vi "Aircraft opCRD Server 0.vi"() -> ()   [LabVIEW 2015]
doc: "This is the FPGA server for the sbRIO for the open-path cavity ring down."
uses:
  Rate.ctl
  <vilib>/Platform/TimedLoop/XDataNode/timing_clust.ctl
  <vilib>/Platform/TimedLoop/XDataNode/nitl_modes.ctl
  <vilib>/Platform/TimedLoop/XDataNode/wakeup.ctl
  <vilib>/rvi/FXPMathLib/FxpDiv/subVIs/nifxpmath_Div_SimConfig.ctl
  <vilib>/rvi/Emulation/niFpgaGetClockAttributes.vi
  <vilib>/rvi/Emulation/niFpgaSctlEmulationGetInTimedLoop.vi
  <vilib>/rvi/Emulation/niFpgaEmulationReportErrorSimple.vi
  <vilib>/rvi/Emulation/niFpgaProcessEmulError.vi
  <vilib>/rvi/eio/common/nirviEmuTemplateMethod_errors.vi
  <vilib>/rvi/Emulation/niFpgaCriticalErrorInLSC.vi
  <vilib>/rvi/FXPMathLib/FxpDiv/simVIs/DllFxpDivTemp_sub.vi
  <vilib>/rvi/interface/RandomDataEmulation/niFpgaRandomDataHandleErrors.vi
  <vilib>/eio/EIONode/EIONode.xnode
  <vilib>/rvi/FXPMathLib/FxpDiv/XNode/nifxpmath_Div.xnode
  <vilib>/rvi/FXPMathLib/FxpMul/XNode/nifxpmath_Multiplier.xnode
  <vilib>/Platform/TimedLoop/XDataNode/XDataNode.xnode
  <vilib>/rvi/DataTransferAndStorage/Container/XNode/niFpgaContainer.xnode
  <vilib>/rvi/interface/RandomDataEmulation/nirviRandomDataFpgaReadWriteTemplate.vi
  <vilib>/Platform/TimedLoop/XDataNode/XDNodeRunTimeDep.lvlib
  <vilib>/rvi/Memory/Memory_Emulation/nirvimemoryFastEmulation.vi
  <vilib>/rvi/Memory/Memory_Emulation/nirvimemoryEmulation.vi
  <vilib>/rvi/FXPMathLib/sim/FxpSim.dll
panel:
  out "CollectData":bool
  in  "max":i32
  in  "InvertLaser?":bool
  in  "LaserOff (us)":u32
  in  "Reverse?":bool
  out "ShipError":bool
  out "EncodeLoop":bool
  out "LaserLoop":bool
  out "ShipLoop":bool
  out "DataLoop":bool
  out "Delay Ticks":u32
  in  "Delay (us)":u16
  out "RequestLaser":bool
  out "Sample Ticks":u32
  in  "Pause Digitizer":bool
  in  "Sample Time (us)":u16
  in  "Rate":T1=3 items=["1 MHz"=20, "2 MHz"=10, "2.5 MHz"=8, "5 MHz"=4, "10 MHz"=2, "20MHz"=1]
  out "LaserOFF?":bool
  in  "Cylce (ticks)":u32=40000
  out "DataRead":bool
  out "dataready":bool
  out "NewData":u16
  out "NumElements":u32
  in  "Stop":bool
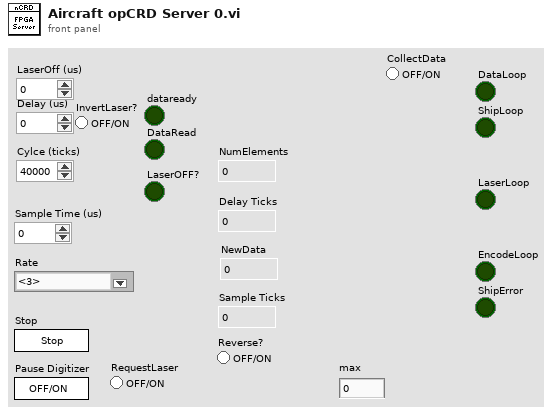
[diagram p1: front panel]
types:
  T1 = typedef "Rate.ctl" = u8
  T2 = cluster{"fixed-point type":fxp<+/-,64,64>, "x+y":fxp<+/-,64,64>, "x+y":fxp<+/-,64,64>, "x+y":fxp<+/-,64,64>, "x+y":fxp<+/-,64,64>, "x+y":fxp<+/-,64,64>, "x+y":fxp<+/-,64,64>}
  T3 = typedef "XDNodeRunTimeDep.lvlib/timing_clust.ctl" = cluster{"Expected End [f-1]":u64, "Actual End [f-1]":u64, "Finished Late? [f-1]":bool, "Expected End [i-1]":u64, "Actual End [i-1]":u64, "Finished Late? [i-1]":bool, "Expected Start [i]":u64, "Actual Start [i]":u64, "Expected Start [f]":u64, "Actual Start [f]":u64, "Source Name":string, "Structure Name":string, "Period":i64, "Deadline":i64, "Offset":i64, "Start":i64, "Priority":i32, "Timeout":i32, "Mode":T4, "Wakeup Reason":T5, "Error":errorcluster, "Source Type":string, "Secondary Source Type":string, "Global End Time":u64, "Global Start Time":u64, "Frame Duration":u64, "Iteration Duration":u64, "Assigned CPU":i32, "I/O Scan Engine Mode":u32}
  T4 = typedef "XDNodeRunTimeDep.lvlib/nitl_modes.ctl" = enum32{"No Change", "Process missed periods, maintain original phase", "Discard missed periods, maintain original phase", "Process missed periods, ignore original phase", "Discard missed periods, ignore original phase"}
  T5 = typedef "XDNodeRunTimeDep.lvlib/wakeup.ctl" = enum32{"Normal", "Aborted", "Asynchronous wakeup", "Timing source error", "Timed loop error", "Timeout"}
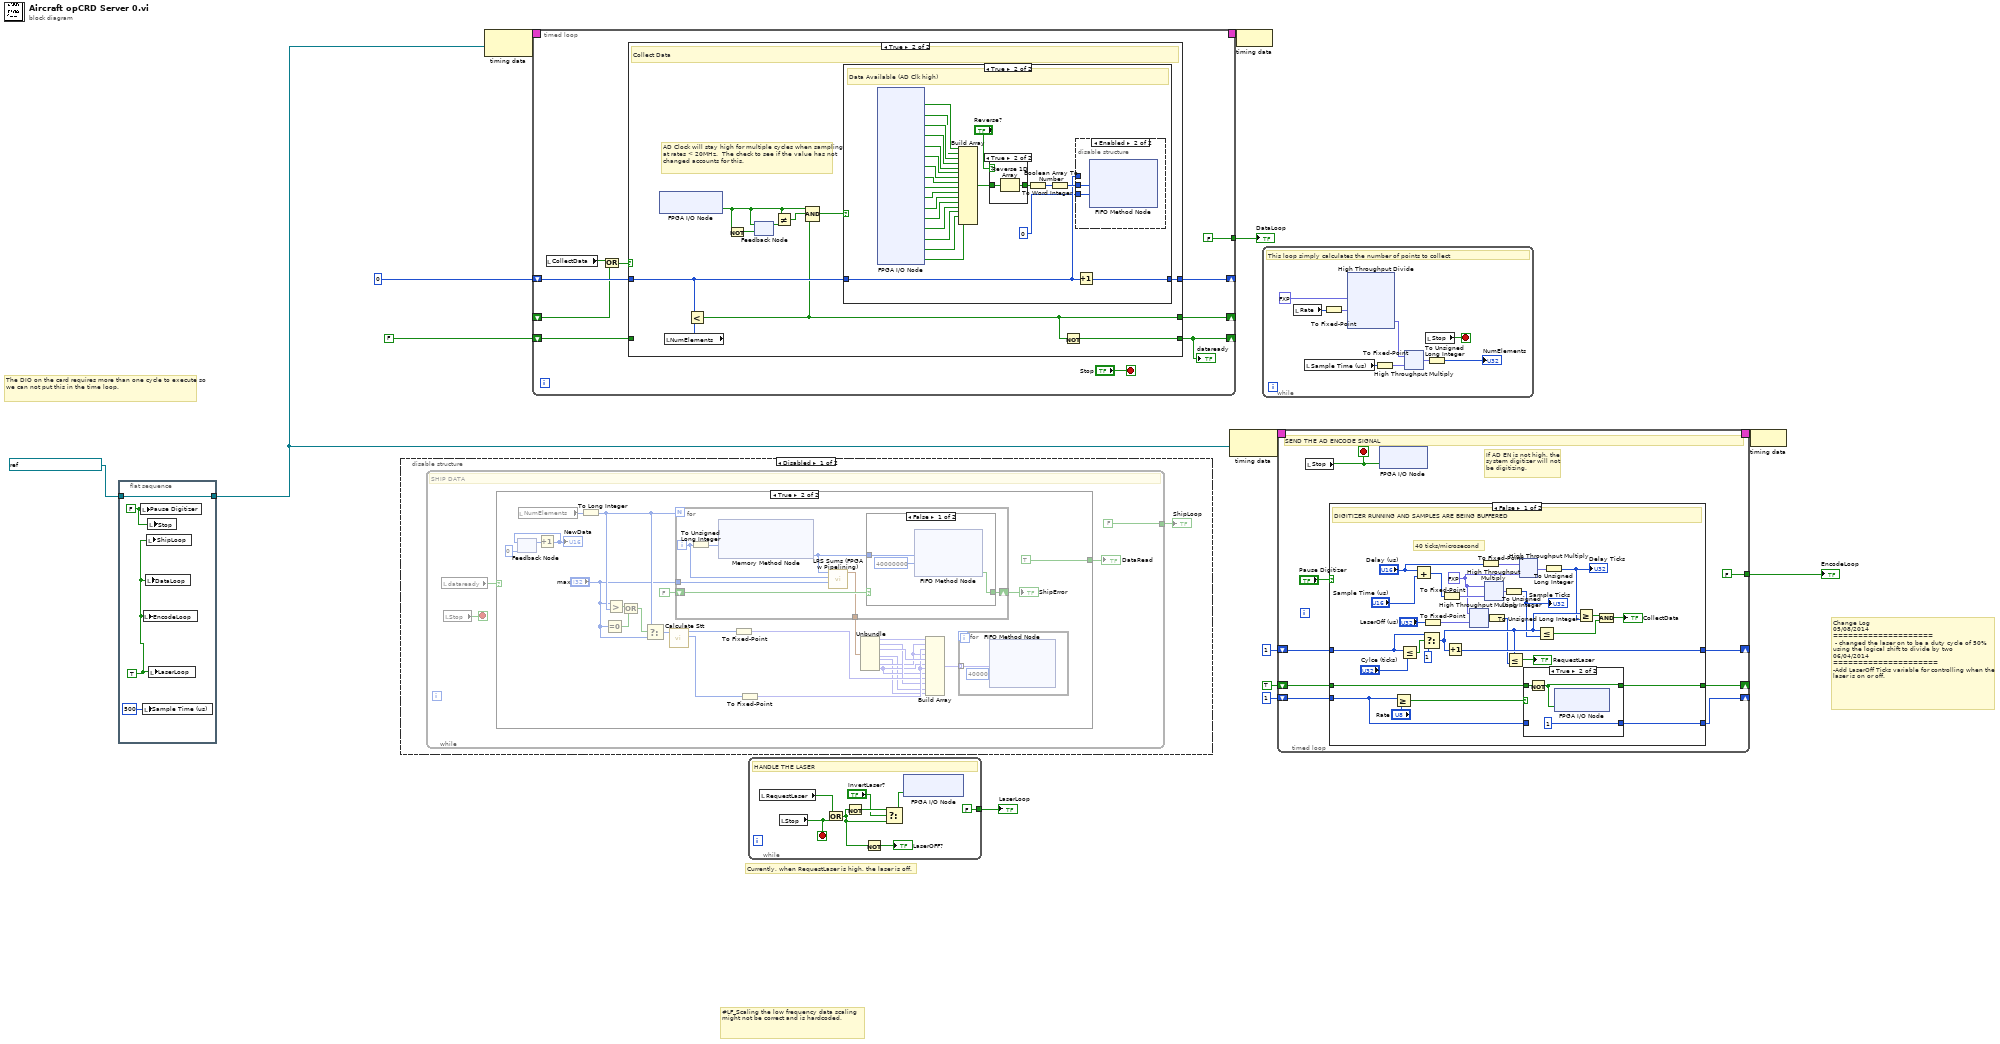
[diagram p0: block diagram]
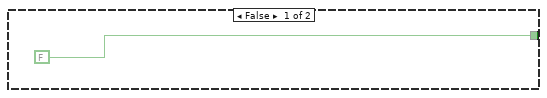
[diagram p2: hidden frame]
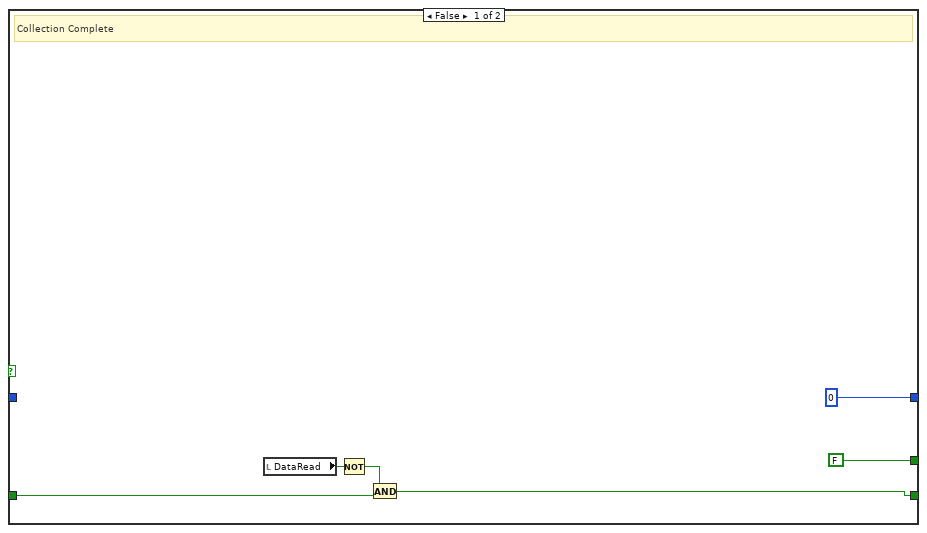
[diagram p5: hidden frame]
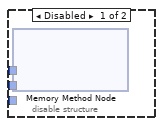
[diagram p7: hidden frame]
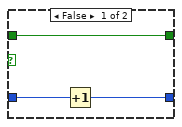
[diagram p9: hidden frame]
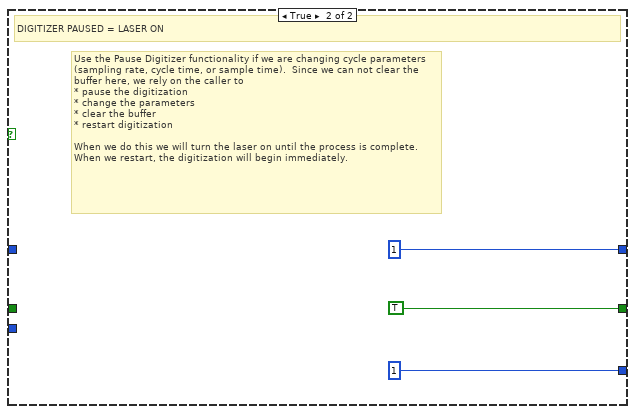
[diagram p10: hidden frame]
diagram:
  # "Change Log\n05/08/2014 \n====================\n - changed the laser on to be a duty cycle of 50% using the logical shift to divide by two\n06/04/2014\n=====================\n-Add LaserOff Ticks variable for controlling when the laser is on or off."
  # "Currently, when RequestLaser is high, the laser is off."
  # "#LF_Scaling the low frequency data scaling might not be correct and is hardcoded."
  # "The DIO on the card requires more than one cycle to execute so we can not put this in the time loop."
  n1 = flat-sequence {
    tunnel: refnum<k21> "40 MHz Onboard Clock" ("Source Name") -> [w18]
    tunnel: [w18] -> w1
    frame #0 {
      w16 = TRUE
      w17 = FALSE ("Pause Digitizer")
      n2 = local write "Pause Digitizer"(w17) -> ()
      n3 = local write "Sample Time (us)"(u16 500 ("Sample Time (us)")) -> ()
      n4 = local write "EncodeLoop"(w16) -> ()
      n5 = local write "DataLoop"(w16) -> ()
      n6 = local write "ShipLoop"(w16) -> ()
      n7 = local write "Stop"(w17) -> ()
      n8 = local write "LaserLoop"(w16) -> ()
    }
  }
  n9 = disable-structure shown="Disabled" {
    frame Disabled {
      n10 = while {
        tunnel: [FALSE] -> w19
        stop <- w23 stop-if-true
        # "SHIP DATA"
        n11 = local read "dataready"() -> (w22:bool)
        n12 = local read "Stop"() -> (w23:bool)
        n13 = case shown="True" w22 {
          tunnel: [FALSE TRUE] -> w21
          frame False {
          }
          frame True {
            n14 = feedback #1(u16 0) -> (w48:u16)
            n15 = local read "NumElements"() -> (w44:u32)
            n16 = Increment(x=w48) -> (x+1=w49:u16)
            "NewData" <- w49
            n17 = feedback-in #1(w49) -> ()
            n18 = To Long Integer(number=w44) -> (32bit integer=w29:i32)
            n19 = Equal To 0?(x="max") -> (x = 0?=w26:bool)
            n20 = Greater?(x="max", y=w29) -> (0:w27:bool)
            n21 = Or(x=w27, y=w26) -> (x .or. y?=w25:bool)
            n22 = Select(t=w29, s=w25, f="max") -> (s? t:f=w43:i32)
            n23 = call "Calculate Stt.vi"("N"=w43) -> ("St"=w41:i64, "Stt"=w42:i64)  [unwired: 9 in]
            n24 = for {
              N: w29 -> [_]
              shift-right: [w56] -> w46
              shift-left: FALSE ("Timed Out?") -> [w55]
              tunnel: [w51] -> w36
              tunnel: "max" -> [w52]
              i -> [w54]
              n25 = To Unsigned Long Integer(number=w54) -> (unsigned 32bit integer=w57:u32)
              n26 = xnode ("Memory Method Node")("Address"=w57) -> ("Data"=w53:i16)  [unwired: 1 in, 1 out]
              n27 = call "LRS Sums (FPGA w Pipelining).vi"("max"=w52, "i"=w54, "DataIn"=w53) -> ("DataOut"=w51:T2)  [unwired: 8 in]
              n28 = case shown="False" w55 {
                selector: w55 -> [_ w61]
                tunnel: w53 -> [w60 _]
                tunnel: [w59 w61] -> w56
                frame False {
                  n29 = xnode ("FIFO Method Node")("Element"=w60, "Timeout"=40000000) -> ("Timed Out?"=w59:bool)  [unwired: 1 in, 1 out]
                }
                frame True {
                }
              }
            }
            "ShipError" <- w46
            n30 = To Fixed-Point(number=w42) -> (fixed-point=w37:fxp<+/-,64,64>)  [unwired: 1 in]
            n31 = To Fixed-Point(number=w41) -> (fixed-point=w38:fxp<+/-,64,64>)  [unwired: 1 in]
            n32 = Unbundle(w36) -> ("fixed-point type"=w40:fxp<+/-,64,64>, "x+y"=w35:fxp<+/-,64,64>, "x+y"=w39:fxp<+/-,64,64>, "x+y"=w32:fxp<+/-,64,64>, "x+y"=w31:fxp<+/-,64,64>, "x+y"=w34:fxp<+/-,64,64>, "x+y"=w33:fxp<+/-,64,64>)
            n33 = Build Array(w40, w34, w38, w34, w39, w33, w38, w33, w37, w35, w32, w31) -> (w30:fxp<+/-,64,64>[])
            n34 = for {
              tunnel: w30 -> [w63] mode=indexing
              n35 = xnode ("FIFO Method Node")("Element"=w63, "Timeout"=40000) -> ()  [unwired: 1 in, 2 out]
            }
          }
        }
        "DataRead" <- w21
      }
      "ShipLoop" <- w19
    }
    frame Enabled {
    }
  }
  n36 = node-c288(w1) -> (w6:T3)
  n37 = timed-loop {
    timing: w6 -> [_]
    timing-out: [_] -> w5
    shift-right: [w71] -> _
    shift-left: u32 0 -> [w70]
    shift-right: [w69] -> _
    shift-left: _ -> [w68]
    shift-right: [w66] -> _
    shift-left: FALSE -> [w65]
    tunnel: [FALSE] -> w2
    stop <- "Stop" stop-if-true
    n38 = local read "CollectData"() -> (w73:bool)
    n39 = Or(x=w73, y=w68) -> (x .or. y?=w72:bool)
    n40 = case shown="True" w72 {
      tunnel: [u32 0 w85] -> w71
      tunnel: w70 -> [_ w86]
      tunnel: [FALSE w81] -> w69
      tunnel: [w74 w80] -> w66
      tunnel: w65 -> [w75 _]
      frame False {
        # "Collection Complete"
        n41 = local read "DataRead"() -> (w77:bool)
        n42 = Not(x=w77) -> (.not. x?=w76:bool)
        n43 = And(x=w76, y=w75) -> (x .and. y?=w74:bool)
      }
      frame True {
        # "AD Clock will stay high for multiple cycles when sampling at rates < 20MHz.  The check to see if the value has not changed accounts for this."
        # "Collect Data"
        n44 = xnode "FPGA I/O Node"() -> ("AD Clock +"=w83:bool)  [unwired: 1 in, 1 out]
        n45 = local read "NumElements"() -> (w89:u32)
        n46 = Less?(x=w86, y=w89) -> (x < y?=w81:bool)
        n47 = Not(x=w83) -> (.not. x?=w87:bool)
        n48 = feedback #2(w87) -> (w88:bool)
        n49 = feedback-in #2(w83) -> ()
        n50 = Not Equal?(x=w83, y=w88) -> (x != y?=w84:bool)
        n51 = Compound Arithmetic op=AND(w83, w84, w81) -> (w82:bool)
        n52 = case shown="True" w82 {
          tunnel: w86 -> [w90 w93]
          tunnel: [w90 w94] -> w85
          frame False {
            # "Waiting (Clk previously high or currently low)"
          }
          frame True {
            # "Data Available (AD Clk high)"
            n53 = xnode "FPGA I/O Node"() -> ("AD0"=w95:bool, "AD1"=w96:bool, "AD2"=w97:bool, "AD3"=w98:bool, "AD4"=w99:bool, "AD5"=w100:bool, "AD6"=w101:bool, "AD7"=w102:bool, "AD8"=w103:bool, "AD9"=w104:bool, "AD10"=w105:bool, "AD11"=w106:bool, "AD12"=w107:bool, "AD13"=w108:bool, "AD14"=w109:bool, "AD15"=w110:bool)  [unwired: 16 in, 16 out]
            n54 = Build Array(w95, w96, w97, w98, w99, w100, w101, w102, w103, w104, w105, w106, w107, w108, w109, w110) -> (w113:bool[])
            n55 = case shown="True" "Reverse?" {
              tunnel: w113 -> [w119 w121]
              tunnel: [w119 w120] -> w114
              frame False {
              }
              frame True {
                n56 = Reverse 1D Array(array=w121) -> (reversed array=w120:bool[])
              }
            }
            n57 = Boolean Array To Number(Boolean array=w114) -> (number=w111:u16)
            n58 = To Word Integer(number=w111) -> (16bit integer=w112:i16)
            n59 = disable-structure shown="Enabled" {
              disable-tunnel: w112 -> [w116 w118]
              disable-tunnel: w93 -> [w115 _]
              disable-tunnel: 0 ("Timeout") -> [_ w117]
              frame Disabled {
                n60 = xnode ("Memory Method Node")("Address"=w115, "Data"=w116) -> ()  [unwired: 1 in, 1 out]
              }
              frame Enabled {
                n61 = xnode ("FIFO Method Node")("Element"=w118, "Timeout"=w117) -> ()  [unwired: 1 in, 2 out]
              }
            }
            n62 = Increment(x=w93) -> (x+1=w94:u32)
          }
        }
        n63 = Not(x=w81) -> (.not. x?=w80:bool)
      }
    }
    "dataready" <- w66
  }
  "DataLoop" <- w2
  n64 = while {
    tunnel: [FALSE] -> w8
    stop <- w130 stop-if-true
    # "HANDLE THE LASER"
    n65 = local read "RequestLaser"() -> (w131:bool)
    n66 = local read "Stop"() -> (w130:bool)
    n67 = Or(x=w131, y=w130) -> (x .or. y?=w125:bool)
    n68 = Not(x=w125) -> (.not. x?=w127:bool)
    n69 = Not(x=w125) -> (.not. x?=→"LaserOFF?":bool)
    n70 = Select(t=w127, s="InvertLaser?", f=w125) -> (s? t:f=w126:bool)
    n71 = xnode "FPGA I/O Node"("Laser Mod"=w126) -> ()  [unwired: 1 in, 1 out]
  }
  "LaserLoop" <- w8
  n72 = node-c288(w1) -> (w14:T3)
  n73 = node-c288(w5) -> ()
  n74 = while {
    stop <- w140 stop-if-true
    # "This loop simply calculates the number of points to collect"
    n75 = local read "Rate"() -> (w136:T1)
    n76 = local read "Sample Time (us)"() -> (w139:u16)
    n77 = To Fixed-Point(number=w136) -> (fixed-point=w135:fxp<+,8,8>)  [unwired: 1 in]
    n78 = xnode "High Throughput Divide"("x"=fxp<+,8,8> 20.0 ("Sample Time (us) 2"), "y"=w135) -> ("x/y"=w134:fxp<+,16,8>)
    n79 = To Fixed-Point(number=w139) -> (fixed-point=w138:fxp<+,16,16>)  [unwired: 1 in]
    n80 = xnode ("High Throughput Multiply")("x"=w134, "y"=w138) -> ("x*y"=w133:fxp<+,32,32>)
    n81 = local read "Stop"() -> (w140:bool)
    n82 = To Unsigned Long Integer(number=w133) -> (unsigned 32bit integer=→"NumElements":u32)
  }
  n83 = timed-loop {
    shift-right: [w172] -> _
    shift-left: TRUE -> [w173]
    timing: w14 -> [_]
    timing-out: [_] -> w13
    shift-right: [w174] -> _
    shift-left: u32 1 -> [w175]
    shift-right: [w171] -> _
    shift-left: u8 1 -> [w170]
    tunnel: [FALSE] -> w7
    stop <- w176 stop-if-true
    # "If AD EN is not high, the system digitizer will not be digitizing."
    # "SEND THE AD ENCODE SIGNAL"
    n84 = local read "Stop"() -> (w176:bool)
    n85 = case shown="False" "Pause Digitizer" {
      tunnel: w175 -> [w189 _]
      tunnel: [w204 u32 1] -> w174
      tunnel: w173 -> [w201 _]
      tunnel: [w200 TRUE ("Element")] -> w172
      tunnel: [w199 u8 1] -> w171
      tunnel: w170 -> [w198 _]
      frame False {
        w185 = fxp<+,8,8> 40.0 ("Sample Time (us) 2")
        # "40 ticks/microsecond"
        # "DIGITIZER RUNNING AND SAMPLES ARE BEING BUFFERED"
        n86 = Greater Or Equal?(x=w198, y="Rate") -> (x >= y?=w202:bool)
        n87 = Less Or Equal?(x=w189, y="Cylce (ticks)") -> (x <= y?=w206:bool)
        n88 = Add(x="Delay (us)", y="Sample Time (us)") -> (x+y=w195:u16)
        n89 = Select(t=w189, s=w206, f=u32 1) -> (s? t:f=w187:u32)
        n90 = To Fixed-Point(number="LaserOff (us)") -> (fixed-point=w183:fxp<+,32,32>)  [unwired: 1 in]
        n91 = To Fixed-Point(number=w195) -> (fixed-point=w196:fxp<+,16,16>)  [unwired: 1 in]
        n92 = Increment(x=w187) -> (x+1=w204:u32)
        n93 = xnode ("High Throughput Multiply")("x"=w185, "y"=w183) -> ("x*y"=w182:fxp<+,32,32>)
        n94 = To Fixed-Point(number="Delay (us)") -> (fixed-point=w192:fxp<+,16,16>)  [unwired: 1 in]
        n95 = xnode ("High Throughput Multiply")("x"=w185, "y"=w196) -> ("x*y"=w197:fxp<+,32,32>)
        n96 = To Unsigned Long Integer(number=w182) -> (unsigned 32bit integer=w181:u32)
        n97 = To Unsigned Long Integer(number=w197) -> (unsigned 32bit integer=w177:u32)
        "Sample Ticks" <- w177
        n98 = Less Or Equal?(x=w187, y=w181) -> (x <= y?=→"RequestLaser":bool)
        n99 = xnode ("High Throughput Multiply")("x"=w192, "y"=w185) -> ("x*y"=w191:fxp<+,32,32>)
        n100 = case shown="True" w202 {
          tunnel: w201 -> [w209 w212]
          tunnel: [w209 w211] -> w200
          tunnel: [w207 u8 1] -> w199
          tunnel: w198 -> [w208 _]
          frame False {
            n101 = Increment(x=w208) -> (x+1=w207:u8)
          }
          frame True {
            n102 = Not(x=w212) -> (.not. x?=w211:bool)
            n103 = xnode "FPGA I/O Node"("ENCODE"=w211) -> ()  [unwired: 1 in, 1 out]
          }
        }
        n104 = Less Or Equal?(x=w187, y=w177) -> (x <= y?=w194:bool)
        n105 = To Unsigned Long Integer(number=w191) -> (unsigned 32bit integer=w178:u32)
        "Delay Ticks" <- w178
        n106 = Greater Or Equal?(x=w187, y=w178) -> (x >= y?=w190:bool)
        n107 = And(x=w190, y=w194) -> (x .and. y?=→"CollectData":bool)
      }
      frame True {
        # "Use the Pause Digitizer functionality if we are changing cycle parameters (sampling rate, cycle time, or sample time).  Since we can not clear the buffer here, we rely on the caller to \n* pause the digitization\n* change the parameters\n* clear the buffer\n* restart digitization\n\nWhen we do this we will turn the laser on until the process is complete. When we restart, the digitization will begin immediately."
        # "DIGITIZER PAUSED = LASER ON"
      }
    }
    n108 = xnode "FPGA I/O Node"("AD EN"=w176) -> ()  [unwired: 1 in, 1 out]
  }
  "EncodeLoop" <- w7
  n109 = node-c288(w13) -> ()
